vi "DesiredBundle2DesiredString.vi"(0 "DesiredParameters":T1, 7 "Controller?":bool) -> (4 "ParameterSet":string)   [LabVIEW 2019]
uses:
  TypeDef/Command Cluster.ctl
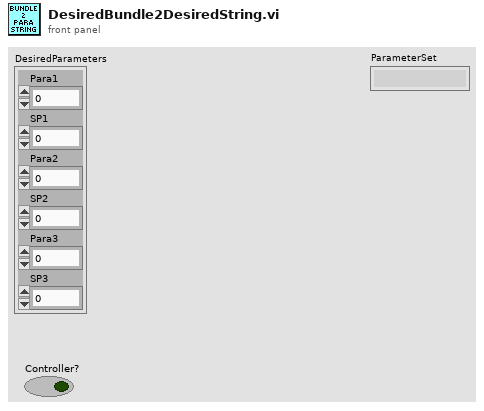
[diagram p1: front panel]
types:
  T1 = typedef "Command Cluster.ctl" = cluster{"Para1":i32, "SP1":dbl, "Para2":i32, "SP2":dbl, "Para3":i32, "SP3":dbl}
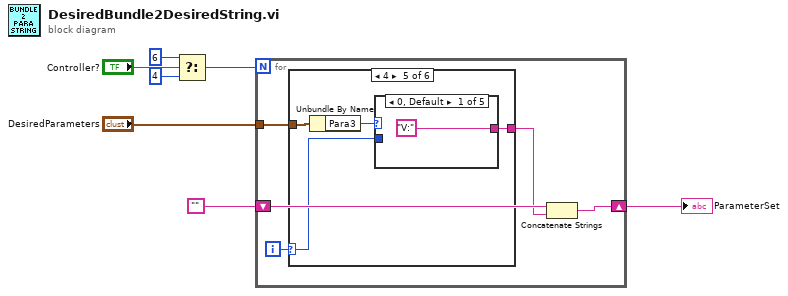
[diagram p0: block diagram]
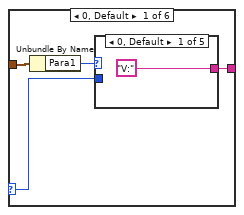
[diagram p2: hidden frame]
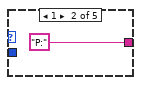
[diagram p3: hidden frame]
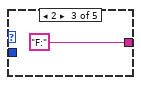
[diagram p4: hidden frame]
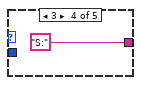
[diagram p5: hidden frame]
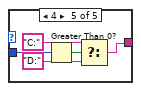
[diagram p6: hidden frame]
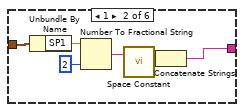
[diagram p7: hidden frame]
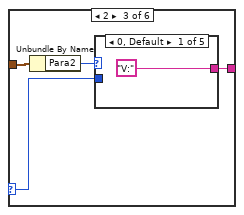
[diagram p8: hidden frame]
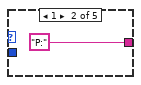
[diagram p9: hidden frame]
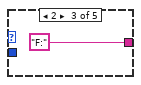
[diagram p10: hidden frame]
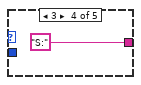
[diagram p11: hidden frame]
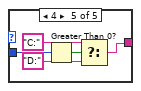
[diagram p12: hidden frame]
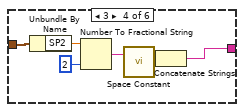
[diagram p13: hidden frame]
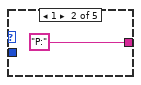
[diagram p14: hidden frame]
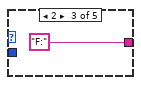
[diagram p15: hidden frame]
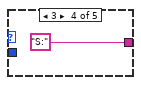
[diagram p16: hidden frame]
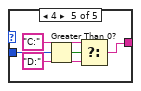
[diagram p17: hidden frame]
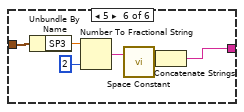
[diagram p18: hidden frame]
diagram:
  n1 = Select(t=6, s="Controller?", f=4) -> (s? t:f=w4:i32)
  n2 = for {
    N: w4 -> [_]
    tunnel: "DesiredParameters" -> [w11]
    shift-right: [w8] -> w1
    shift-left: "" -> [w10]
    i -> [w12]
    n3 = case shown="4" w12 {
      selector: w12 -> [w14 _ w32 _ w51 _]
      tunnel: w11 -> [w16 w31 w35 w50 w54 w69]
      tunnel: [w13 w26 w33 w45 w52 w64] -> w9
      frame 0, Default {
        n4 = Unbundle By Name(w16) -> ("Para1"=w15:i32)
        n5 = case shown="0, Default" w15 {
          tunnel: ["V:" "P:" "F:" "S:" w21] -> w13
          tunnel: w14 -> [_ _ _ _ w25]
          frame 0, Default {
          }
          frame 1 {
          }
          frame 2 {
          }
          frame 3 {
          }
          frame 4 {
            n6 = Greater Than 0?(x=w25) -> (x > 0?=w24:bool)
            n7 = Select(t="C:", s=w24, f="D:") -> (s? t:f=w21:string)
          }
        }
      }
      frame 1 {
        n8 = Unbundle By Name(w31) -> ("SP1"=w30:dbl)
        n9 = Number To Fractional String(number=w30, precision (6)=i16 2) -> (F-format string=w28:string)  [unwired: 2 in]
        n10 = call <vilib>:"Space Constant.vi"() -> ("String"=w27:string)
        n11 = Concatenate Strings(w28, w27) -> (w26:string)
      }
      frame 2 {
        n12 = Unbundle By Name(w35) -> ("Para2"=w34:i32)
        n13 = case shown="0, Default" w34 {
          tunnel: ["V:" "P:" "F:" "S:" w40] -> w33
          tunnel: w32 -> [_ _ _ _ w44]
          frame 0, Default {
          }
          frame 1 {
          }
          frame 2 {
          }
          frame 3 {
          }
          frame 4 {
            n14 = Greater Than 0?(x=w44) -> (x > 0?=w43:bool)
            n15 = Select(t="C:", s=w43, f="D:") -> (s? t:f=w40:string)
          }
        }
      }
      frame 3 {
        n16 = Unbundle By Name(w50) -> ("SP2"=w48:dbl)
        n17 = Number To Fractional String(number=w48, precision (6)=i16 2) -> (F-format string=w46:string)  [unwired: 2 in]
        n18 = call <vilib>:"Space Constant.vi"() -> ("String"=w47:string)
        n19 = Concatenate Strings(w46, w47) -> (w45:string)
      }
      frame 4 {
        n20 = Unbundle By Name(w54) -> ("Para3"=w53:i32)
        n21 = case shown="0, Default" w53 {
          tunnel: ["V:" "P:" "F:" "S:" w59] -> w52
          tunnel: w51 -> [_ _ _ _ w63]
          frame 0, Default {
          }
          frame 1 {
          }
          frame 2 {
          }
          frame 3 {
          }
          frame 4 {
            n22 = Greater Than 0?(x=w63) -> (x > 0?=w62:bool)
            n23 = Select(t="C:", s=w62, f="D:") -> (s? t:f=w59:string)
          }
        }
      }
      frame 5 {
        n24 = Unbundle By Name(w69) -> ("SP3"=w67:dbl)
        n25 = Number To Fractional String(number=w67, precision (6)=i16 2) -> (F-format string=w65:string)  [unwired: 2 in]
        n26 = call <vilib>:"Space Constant.vi"() -> ("String"=w66:string)
        n27 = Concatenate Strings(w65, w66) -> (w64:string)
      }
    }
    n28 = Concatenate Strings(w10, w9) -> (w8:string)
  }
  "ParameterSet" <- w1
